vi "SetName.vi"(8 "ErrorIn":errorcluster, 10 "Name":string, 11 "ReferenceIn":refnum<class "TAFBaseGUI.lvclass">) -> (0 "ErrorOut":errorcluster, 3 "ReferenceOut":refnum<class "TAFBaseGUI.lvclass">)   [LabVIEW 2021, in "TAFBaseGUI.lvclass"]
uses:
  TAFBaseGUI.lvclass
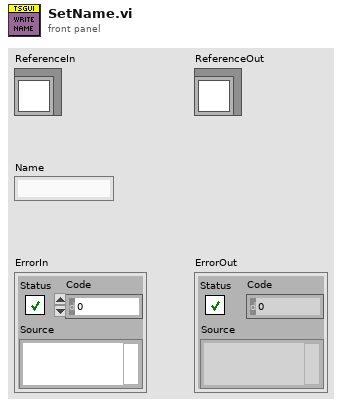
[diagram p1: front panel]
types:
  T1 = typedef "TAFBaseGUI.lvclass/ObjectAttributes.ctl" = cluster{"Name":string, "FPVIRef":refnum<vi>}
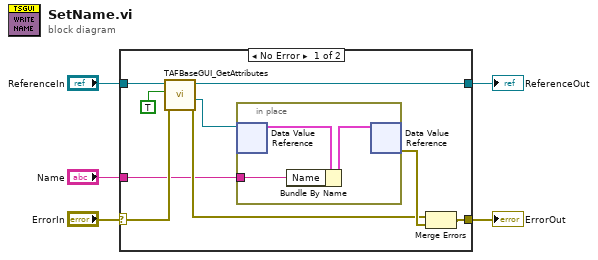
[diagram p0: block diagram]
diagram:
  n1 = case shown="No Error" "ErrorIn" {
    selector: "ErrorIn" -> [w12 w19]
    tunnel: [w13 w19] -> w4
    tunnel: [w8 w18] -> w2
    tunnel: "ReferenceIn" -> [w9 w18]
    tunnel: "Name" -> [w10 _]
    frame No Error {
      n2 = call "TAFBaseGUI_GetAttributes.vi"("ErrorIn"=w12, "OnlyGetDvrReference(False)"=TRUE, "ReferenceIn"=w9) -> ("ErrorOut"=w11:errorcluster, "DataRef"=w7:refnum<data-value>, "ReferenceOut"=w8:refnum<class "TAFBaseGUI.lvclass">)  [unwired: 5 in, 1 out]
      n3 = in-place {
        in-place-border: w10 -> [w17]
        n4 = in-place-dvr #1(w7) -> (w16:T1)  [unwired: 1 out]
        n5 = Bundle By Name(cluster=w16, "Name"=w17) -> (w15:T1)
        n6 = in-place-dvr #1(w15) -> (w14:errorcluster)  [unwired: 1 out]
      }
      n7 = Merge Errors(w11, w14) -> (w13:errorcluster)
    }
    frame Error {
    }
  }
  "ErrorOut" <- w4
  "ReferenceOut" <- w2
